vi "Waveform data class VI - add total displacement.vi"(8 "error in (no error)":errorcluster, 10 "Total displacement":dbl, 11 "Waveform data in":refnum<class "Waveform data.lvclass">) -> (0 "error out":errorcluster, 3 "Waveform data out":refnum<class "Waveform data.lvclass">)   [LabVIEW 2010, in "Waveform data.lvclass"]
uses:
  Waveform data.lvclass
  Waveform data.lvclass/Waveform data.ctl
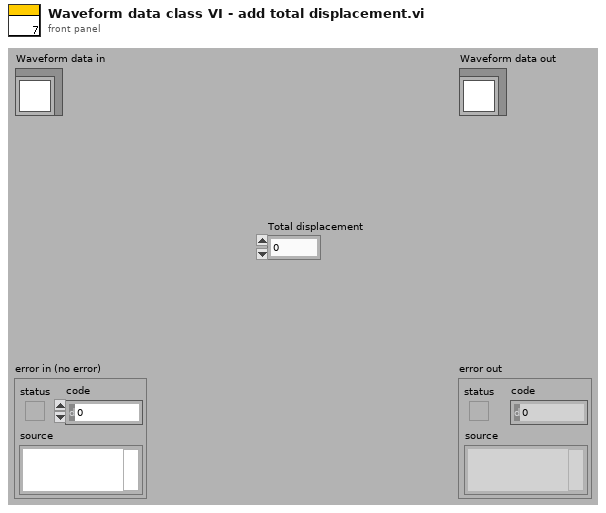
[diagram p1: front panel]
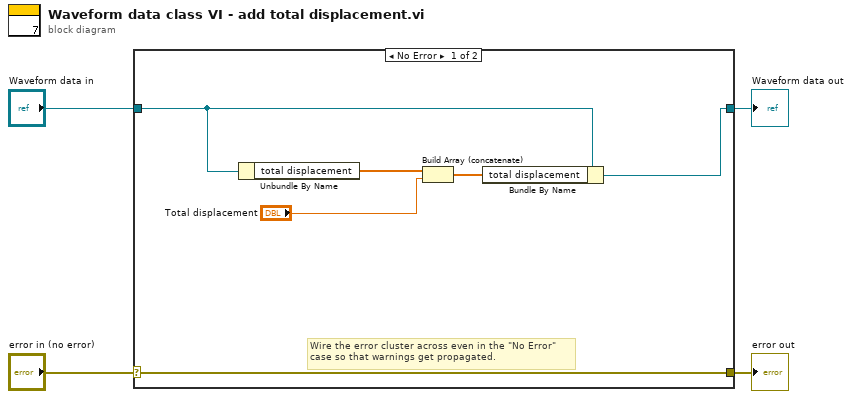
[diagram p0: block diagram]
diagram:
  n1 = case shown="No Error" "error in (no error)" {
    selector: "error in (no error)" -> [w10 w12]
    tunnel: [w10 w12] -> w3
    tunnel: [w6 w11] -> w1
    tunnel: "Waveform data in" -> [w7 w11]
    frame No Error {
      # "Wire the error cluster across even in the \"No Error\"\ncase so that warnings get propagated."
      n2 = Unbundle By Name(w7) -> ("total displacement"=w8:dbl[])
      n3 = Build Array (concatenate)(w8, "Total displacement") -> (w5:dbl[])
      n4 = Bundle By Name(cluster=w7, "total displacement"=w5) -> (w6:refnum<class "Waveform data.lvclass">)
    }
    frame Error {
    }
  }
  "error out" <- w3
  "Waveform data out" <- w1
